vi "Write Authentication Token.vi"(8 "error in (no error)":errorcluster, 10 "Authentication Token":string, 11 "Strava curl in":refnum<class "Strava curl.lvclass">) -> (0 "error out":errorcluster, 3 "Strava curl out":refnum<class "Strava curl.lvclass">)   [LabVIEW 2020, in "Strava curl.lvclass"]
uses:
  Strava curl.lvclass
  Strava curl.lvclass/Strava curl.ctl
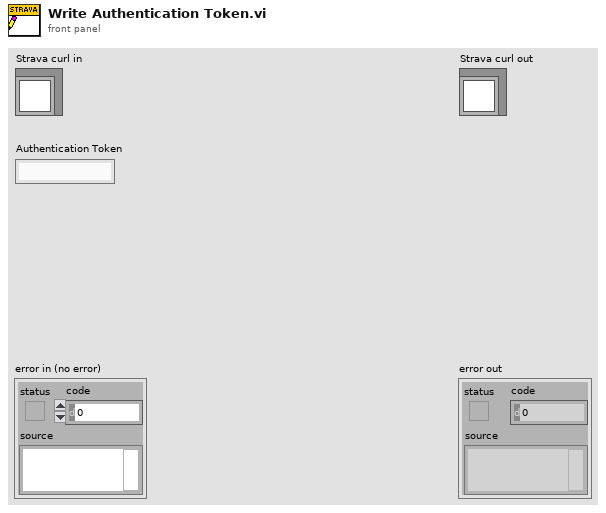
[diagram p1: front panel]
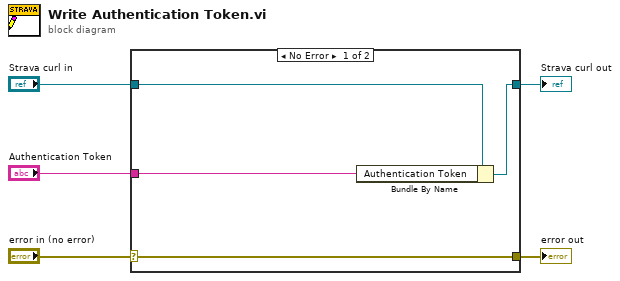
[diagram p0: block diagram]
diagram:
  n1 = case shown="No Error" "error in (no error)" {
    selector: "error in (no error)" -> [w9 w10]
    tunnel: [w9 w10] -> w4
    tunnel: [w7 w11] -> w2
    tunnel: "Strava curl in" -> [w8 w11]
    tunnel: "Authentication Token" -> [w6 _]
    frame No Error {
      n2 = Bundle By Name(cluster=w8, "Authentication Token"=w6) -> (w7:refnum<class "Strava curl.lvclass">)
    }
    frame Error {
    }
  }
  "error out" <- w4
  "Strava curl out" <- w2
